vi "hdf5(SubVI).vi"(0 "Refnum in":refnum<k21>, 1 "VISA Refnum in":refnum<visa-resource-name>="GPIB0::19::INSTR", 2 "appended path":path, 3 "Max Voltage":dbl, 4 "error out 3":errorcluster, 5 "f":i32, 6 "SampClk.Rate":dbl, 7 "error in (no error)":errorcluster, 8 "FPGA VI Reference Out":refnum<k20>, 9 "drive_amplitude":dbl, 10 "task in":refnum<k21>, 13 "drive_freq":dbl, 17 "volt_div":dbl) -> (14 "task out 4":refnum<k21>, 16 "Array":dbl[][](array[numeric]), 18 "CC read error":errorcluster={"status"=FALSE, "code"=1073676294, "source"="VISA Read in datataker.vi"}, 20 "Refnum out":refnum<k21>, 21 "error out":errorcluster, 22 "error out 4":errorcluster, 23 "error out 2":errorcluster, 24 "Pirani pressure (mbar)":string, 25 "CC pressure (mbar)":string="2.4e", 26 "Temps (C):":dbl[](array[numeric])=[20.9, 21.3], 27 "error out":errorcluster={"status"=FALSE, "code"=1073676294, "source"="VISA Read in datataker.vi"})   [LabVIEW 2013]
uses:
  <vilib>/addons/h5labview2/file/H5Fmode.ctl
  <vilib>/DAQmx/read.llb/DAQmx Read (Analog 2D DBL NChan NSamp).vi
  <vilib>/DAQmx/miscellaneous.llb/DAQmx Fill In Error Info.vi
  <vilib>/Utility/error.llb/Error Cluster From Error Code.vi
  <vilib>/rvi/errors/niLvFpgaAdjustHostInterfaceError.vi
  <vilib>/addons/h5labview2/base/lib_path.vi
  <vilib>/addons/h5labview2/base/H5Equery.vi
  <vilib>/rvi/interface/nirviReadWriteControl/nirviReadWriteControl.xnode
  fpga/MultiChannelFeed_FPGATarget2_feedbackcooling(_T5hmXv3JUos.lvbitx
  <vilib>/addons/h5labview2/dataset/H5Dwrite.llb/H5Dwrite.xnode
  <vilib>/addons/h5labview2/attrib/H5Awrite.llb/H5Awrite.xnode
  <vilib>/addons/h5labview2/file/H5F.lvlib
  <vilib>/addons/h5labview2/group/H5G.lvlib
  NiFpgaLv.dll
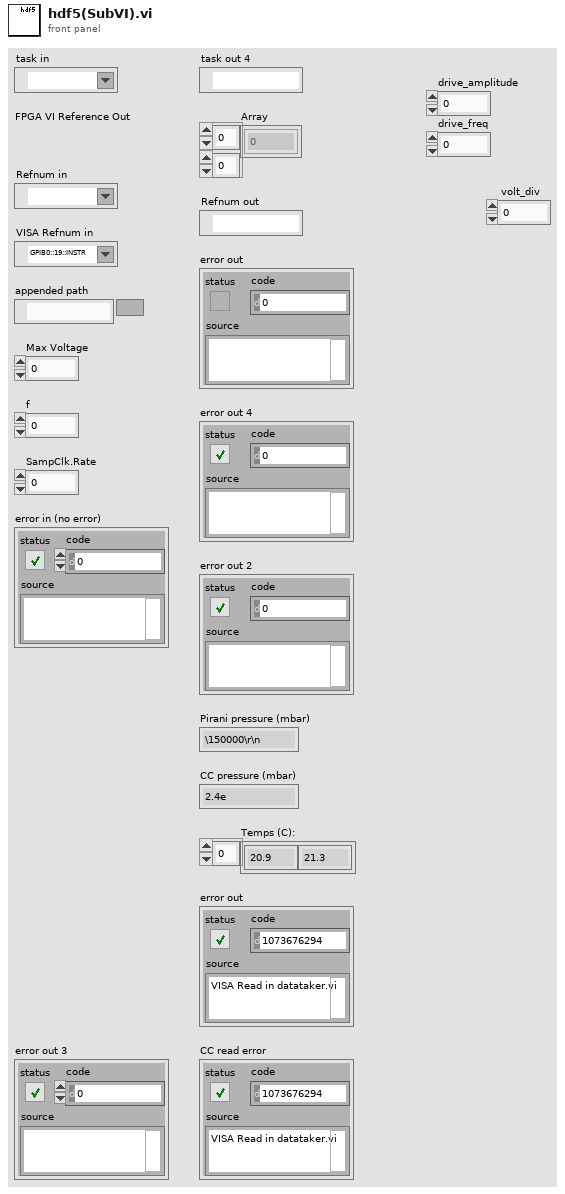
[diagram p1: front panel]
types:
  T1 = typedef "H5F.lvlib/H5Fmode.ctl" = enum16{"read-only", "read-write", "overwrite", "create new", "open or create"}
  T2 = typedef "hid_t.ctl" = i32
  T3 = cluster{"pg 0":fxp<+/-,32,16>, "dg 0":fxp<+/-,32,16>, "pg 1":fxp<+/-,32,16>, "dg 1":fxp<+/-,32,16>, "pg 2":fxp<+/-,32,16>, "dg 2":fxp<+/-,32,16>, "Dc offset 0":fxp<+/-,32,16>, "Dc offset 1":fxp<+/-,32,16>, "Dc offset 2":fxp<+/-,32,16>}
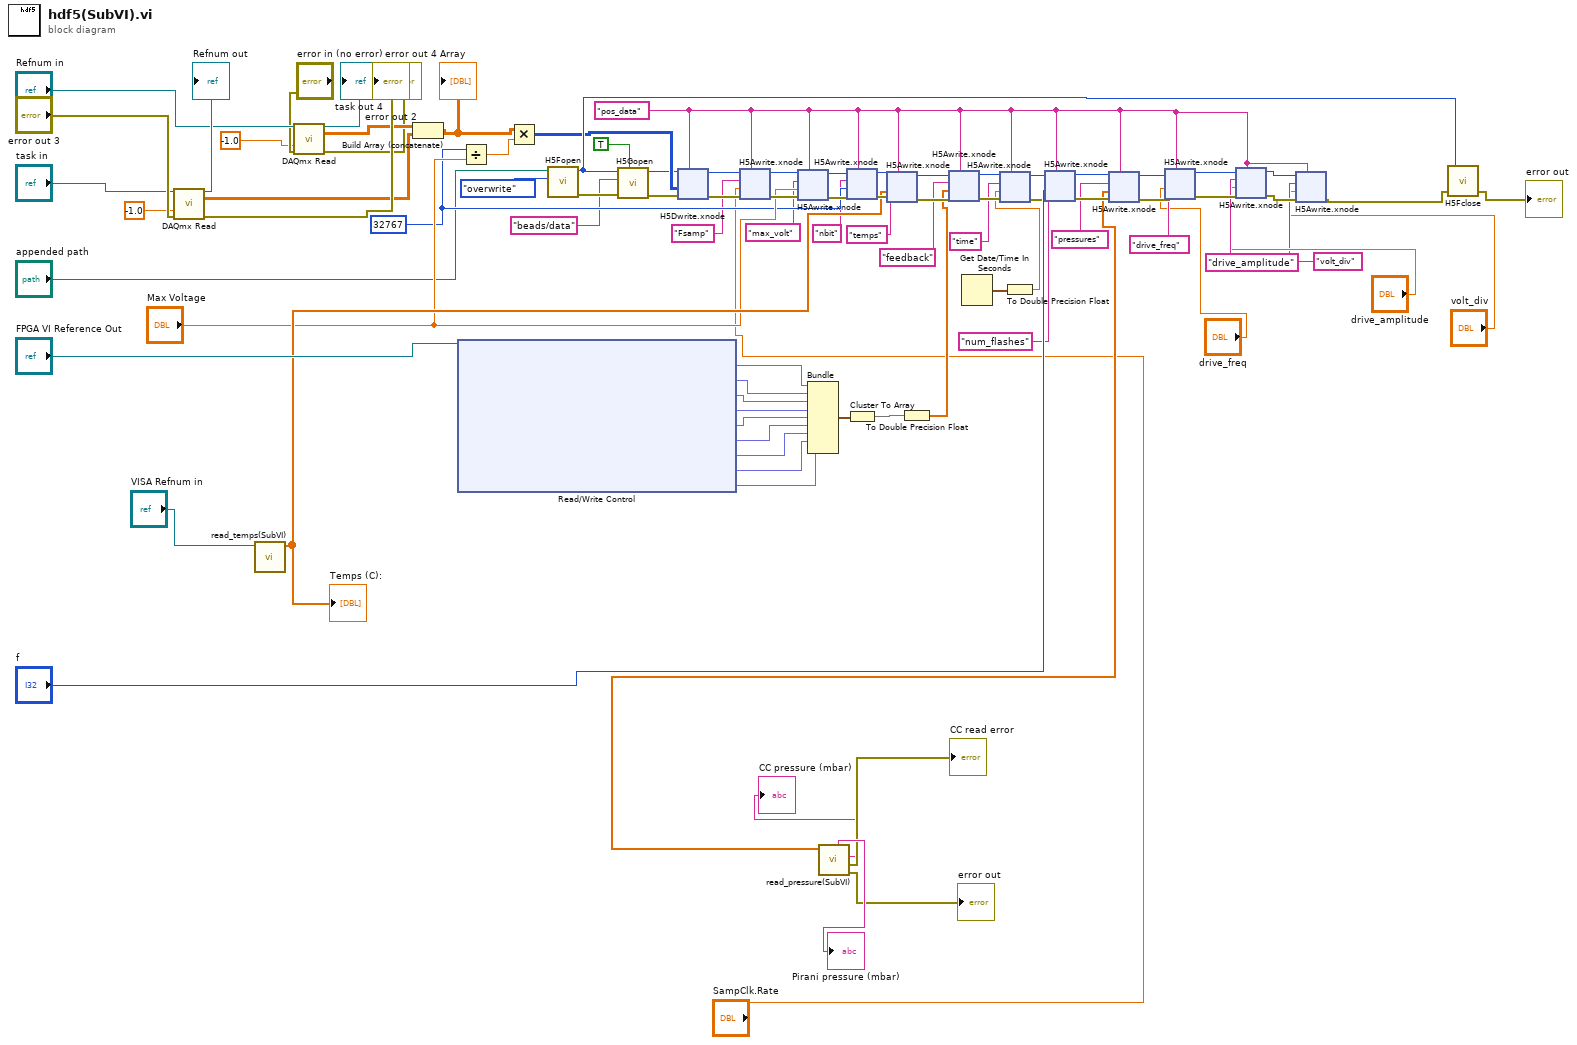
[diagram p0: block diagram]
diagram:
  w34 = i16 32767 ("y")
  w1 = "pos_data" ("dataset name")
  n1 = call-poly <vilib>:"DAQmx Read.vi"("task/channels in"="task in", "timeout"=-1.0, "error in"="error out 3") -> ("task out"=→"Refnum out":refnum<k21>, "data"=w75:dbl[][], "error out"=→"error out 2":errorcluster)  [unwired: 10 in]
  n2 = call "read_temps(SubVI).vi"("VISA Refnum in"="VISA Refnum in") -> ("Array"=w56:dbl[])  [unwired: 10 in]
  "Temps (C):" <- w56
  n3 = call-poly <vilib>:"DAQmx Read.vi"("task/channels in"="Refnum in", "timeout"=-1.0, "error in"="error in (no error)") -> ("task out"=→"task out 4":refnum<k21>, "data"=w74:dbl[][], "error out"=→"error out 4":errorcluster)  [unwired: 10 in]
  n4 = Build Array (concatenate)(w74, w75) -> (w76:dbl[][])
  "Array" <- w76
  n5 = xnode "Read/Write Control"("FPGA VI Reference In"="FPGA VI Reference Out") -> ("pg 0"=w42:fxp<+/-,32,16>, "dg 0"=w43:fxp<+/-,32,16>, "pg 1"=w44:fxp<+/-,32,16>, "dg 1"=w45:fxp<+/-,32,16>, "pg 2"=w46:fxp<+/-,32,16>, "dg 2"=w47:fxp<+/-,32,16>, "Dc offset 0"=w48:fxp<+/-,32,16>, "Dc offset 1"=w49:fxp<+/-,32,16>, "Dc offset 2"=w50:fxp<+/-,32,16>)  [unwired: 1 in, 2 out]
  n6 = Divide(x=w34, y="Max Voltage") -> (x/y=w33:dbl)
  n7 = Multiply(x=w76, y=w33) -> (x*y=w36:i16[][])
  n8 = call <vilib>:"H5Fopen.vi"("mode (read-only)"=H5Fmode."overwrite", "path"="appended path") -> ("error out"=w60:errorcluster, "ref out"=w68:T2)  [unwired: 4 in]
  n9 = call <vilib>:"H5Gopen.vi"("create? (F)"=TRUE, "error in (no error)"=w60, "name"="beads/data", "ref in"=w68) -> ("error out"=w61:errorcluster, "group out"=w20:T2)  [unwired: 3 in]
  n10 = xnode "H5Dwrite.xnode"("dataset name"=w1, "error in (no error)"=w61, "data"=w36, "ref in"=w20) -> ("error out"=w62:errorcluster, "ref out"=w21:i32)  [unwired: 3 in, 1 out]
  n11 = xnode "H5Awrite.xnode"("object name"=w1, "error in (no error)"=w62, "data"="SampClk.Rate", "attrib name"="Fsamp", "ref in"=w21) -> ("error out"=w63:errorcluster, "ref out"=w29:i32)  [unwired: 2 in, 1 out]
  n12 = xnode "H5Awrite.xnode"("object name"=w1, "error in (no error)"=w63, "data"="Max Voltage", "attrib name"="max_volt", "ref in"=w29) -> ("error out"=w64:errorcluster, "ref out"=w31:i32)  [unwired: 2 in, 1 out]
  n13 = Bundle("pg 0"=w42, "dg 0"=w43, "pg 1"=w44, "dg 1"=w45, "pg 2"=w46, "dg 2"=w47, "Dc offset 0"=w48, "Dc offset 1"=w49, "Dc offset 2"=w50) -> (w41:T3)  [unwired: 1 in]
  n14 = call "read_pressure(SubVI).vi"() -> ("error out"=→"error out":errorcluster, "CC read error"=→"CC read error":errorcluster, "CC pressure (mbar)"=→"CC pressure (mbar)":string, "Array"=w82:dbl[], "Pirani pressure (mbar)"=→"Pirani pressure (mbar)":string)  [unwired: 7 in]
  n15 = xnode "H5Awrite.xnode"("object name"=w1, "error in (no error)"=w64, "data"=w34, "attrib name"="nbit", "ref in"=w31) -> ("error out"=w65:errorcluster, "ref out"=w38:i32)  [unwired: 2 in, 1 out]
  n16 = Cluster To Array(cluster=w41) -> (array=w51:fxp<+/-,32,16>[])
  n17 = xnode "H5Awrite.xnode"("object name"=w1, "error in (no error)"=w65, "data"=w56, "attrib name"="temps", "ref in"=w38) -> ("error out"=w66:errorcluster, "ref out"=w39:i32)  [unwired: 2 in, 1 out]
  n18 = To Double Precision Float(number=w51) -> (double precision float=w52:dbl[])
  n19 = xnode "H5Awrite.xnode"("object name"=w1, "error in (no error)"=w66, "data"=w52, "attrib name"="feedback", "ref in"=w39) -> ("error out"=w67:errorcluster, "ref out"=w54:i32)  [unwired: 2 in, 1 out]
  n20 = Get Date/Time In Seconds() -> (seconds since 1Jan1904=w58:timestamp)
  n21 = To Double Precision Float(number=w58) -> (double precision float=w59:dbl)
  n22 = xnode "H5Awrite.xnode"("object name"=w1, "error in (no error)"=w67, "data"=w59, "attrib name"="time", "ref in"=w54) -> ("error out"=w70:errorcluster, "ref out"=w69:i32)  [unwired: 2 in, 1 out]
  n23 = xnode "H5Awrite.xnode"("object name"=w1, "error in (no error)"=w70, "data"="f", "attrib name"="num_flashes", "ref in"=w69) -> ("error out"=w83:errorcluster, "ref out"=w81:i32)  [unwired: 2 in, 1 out]
  n24 = xnode "H5Awrite.xnode"("object name"=w1, "error in (no error)"=w83, "data"=w82, "attrib name"="pressures", "ref in"=w81) -> ("error out"=w15:errorcluster, "ref out"=w11:i32)  [unwired: 2 in, 1 out]
  n25 = xnode "H5Awrite.xnode"("object name"=w1, "error in (no error)"=w15, "data"="drive_freq", "attrib name"="drive_freq", "ref in"=w11) -> ("error out"=w14:errorcluster, "ref out"=w10:i32)  [unwired: 2 in, 1 out]
  n26 = xnode "H5Awrite.xnode"("object name"=w1, "error in (no error)"=w14, "data"="drive_amplitude", "attrib name"="drive_amplitude", "ref in"=w10) -> ("error out"=w6:errorcluster, "ref out"=w5:i32)  [unwired: 2 in, 1 out]
  n27 = xnode "H5Awrite.xnode"("object name"=w1, "error in (no error)"=w6, "data"="volt_div", "attrib name"="volt_div", "ref in"=w5) -> ("error out"=w4:errorcluster)  [unwired: 2 in, 2 out]
  n28 = call <vilib>:"H5Fclose.vi"("error in (no error)"=w4, "ref"=w68) -> ("error out"=→"error out":errorcluster)  [unwired: 3 in]
